vi "DAC Run.vi"(8 "error in":errorcluster, 11 "DAC LN2 Temp in":refnum<class "DAC LN2 Temp.lvclass">) -> (0 "error out":errorcluster, 3 "DAC LN2 Temp out":refnum<class "DAC LN2 Temp.lvclass">)   [LabVIEW 2019, in "DAC.lvlib" / "DAC LN2 Temp.lvclass"]
uses:
  DAC LN2 Temp.lvclass
  DAC.lvclass
  Results/Results Method.ctl
  Results/Results.lvlib
  Results/HTS Results/HTS Results.lvclass
  <vilib>/DAQmx/read.llb/DAQmx Read (Analog DBL 1Chan 1Samp).vi
  C:/Users/krio/Documents/LV_Projects/test-stand/App/DAC/DAC.lvclass
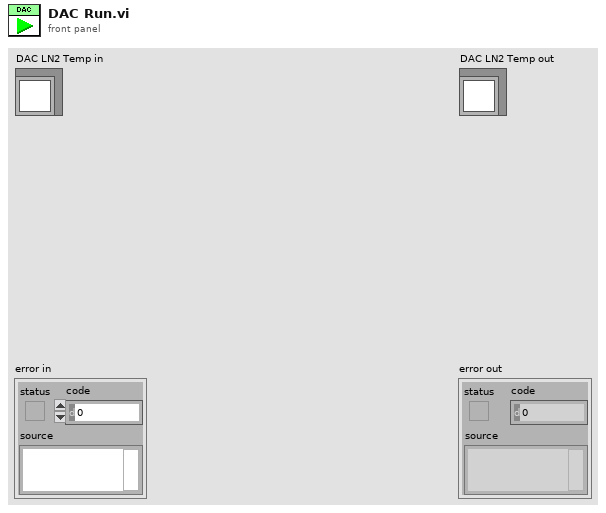
[diagram p1: front panel]
types:
  T1 = typedef "Results.lvlib/Results Method.ctl" = enum16{"Get", "Set"}
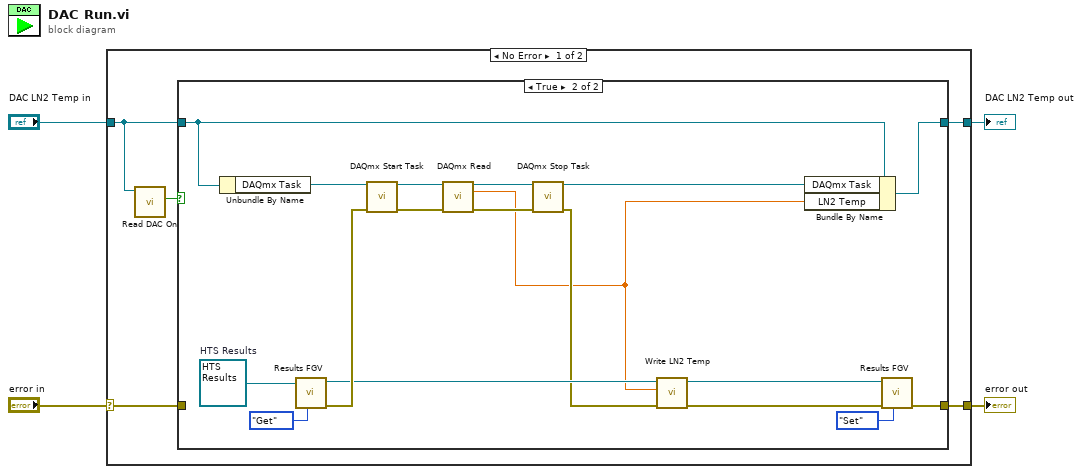
[diagram p0: block diagram]
diagram:
  n1 = case shown="No Error" "error in" {
    selector: "error in" -> [w7 w31]
    tunnel: [w6 w31] -> w2
    tunnel: [w8 w30] -> w1
    tunnel: "DAC LN2 Temp in" -> [w5 w30]
    frame No Error {
      n2 = call "Read DAC On.vi"("DAC in"=w5) -> ("DAC On"=w9:bool)  [unwired: 8 in, 2 out]
      n3 = case shown="True" w9 {
        tunnel: w5 -> [w11 w25]
        tunnel: [w11 w18] -> w8
        tunnel: w7 -> [w10 _]
        tunnel: [w10 w17] -> w6
        frame False {
        }
        frame True {
          w24 = refnum<class "HTS Results.lvclass"> refnum  # HTS Results
          n4 = Unbundle By Name(w25) -> ("DAQmx Task"=w29:refnum<k21>)
          n5 = call-dynamic "Results FGV.vi"("Method"=Results_Method."Get", "HTS Results in"=w24) -> ("error out"=w21:errorcluster, "HTS Results out"=w16:refnum<class "HTS Results.lvclass">)  [unwired: 8 in]
          n6 = call <vilib>:"DAQmx Start Task.vi"("task/channels in"=w29, "error in"=w21) -> ("task out"=w28:refnum<k21>, "error out"=w27:errorcluster)  [unwired: 12 in]
          n7 = call-poly <vilib>:"DAQmx Read.vi"("task/channels in"=w28, "error in"=w27) -> ("task out"=w19:refnum<k21>, "data"=w12:dbl, "error out"=w26:errorcluster)  [unwired: 11 in]
          n8 = call <vilib>:"DAQmx Stop Task.vi"("task/channels in"=w19, "error in"=w26) -> ("task out"=w20:refnum<k21>, "error out"=w13:errorcluster)  [unwired: 12 in]
          n9 = call "Write LN2 Temp.vi"("error in (no error)"=w13, "LN2 Temp"=w12, "HTS Results in"=w16) -> ("error out"=w14:errorcluster, "HTS Results out"=w15:refnum<class "HTS Results.lvclass">)  [unwired: 7 in]
          n10 = Bundle By Name(cluster=w25, "DAQmx Task"=w20, "LN2 Temp"=w12) -> (w18:refnum<class "DAC LN2 Temp.lvclass">)
          n11 = call-dynamic "Results FGV.vi"("Method"=Results_Method."Set", "error in"=w14, "HTS Results in"=w15) -> ("error out"=w17:errorcluster)  [unwired: 7 in, 1 out]
        }
      }
    }
    frame Error {
    }
  }
  "error out" <- w2
  "DAC LN2 Temp out" <- w1
